vi "GEA2 Add ESC Char.vi"(5 "Message":u8[](array[numeric]) format="%.0x") -> (6 "Message Out":u8[](array[numeric]))   [LabVIEW 2009]
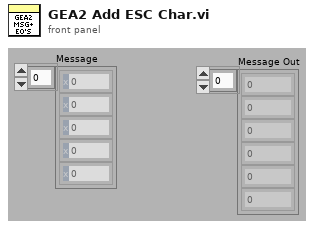
[diagram p1: front panel]
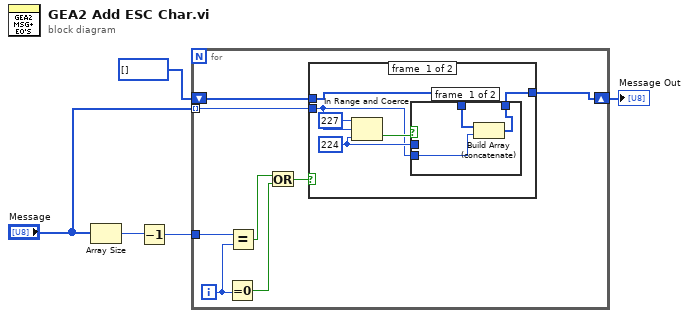
[diagram p0: block diagram]
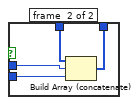
[diagram p2: hidden frame]
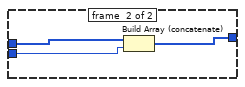
[diagram p3: hidden frame]
diagram:
  n1 = Array Size(array="Message") -> (size(s)=w5:i32)
  n2 = Decrement(x=w5) -> (x-1=w4:i32)
  n3 = for {
    tunnel: w4 -> [w12]
    tunnel: "Message" -> [w8] mode=indexing
    shift-right: [w6] -> w1
    shift-left: u8[] [] -> [w7]
    i -> [w13]
    n4 = Equal To 0?(x=w13) -> (x = 0?=w10:bool)
    n5 = Equal?(x=w12, y=w13) -> (x = y?=w9:bool)
    n6 = Or(x=w9, y=w10) -> (x .or. y?=w11:bool)
    n7 = case shown="False" w11 {
      tunnel: w8 -> [w15 w28]
      tunnel: [w14 w27] -> w6
      tunnel: w7 -> [w17 w29]
      frame #0 {
        w16 = u8 224 ("upper limit")
        n8 = In Range and Coerce(upper limit=u8 227, x=w15, lower limit=w16) -> (In Range?=w18:bool)  [unwired: 1 out]
        n9 = case shown="False" w18 {
          tunnel: w17 -> [w22 w26]
          tunnel: w16 -> [_ w25]
          tunnel: w15 -> [w20 w24]
          tunnel: [w21 w23] -> w14
          frame #0 {
            n10 = Build Array (concatenate)(w22, w20) -> (w21:u8[])
          }
          frame #1 {
            n11 = Build Array (concatenate)(w26, w25, w24) -> (w23:u8[])
          }
        }
      }
      frame #1 {
        n12 = Build Array (concatenate)(w29, w28) -> (w27:u8[])
      }
    }
  }
  "Message Out" <- w1
